vi "signal2.vi"() -> ()   [LabVIEW 2021]
panel:
  in  "?":bool
  out "Waveform Graph":dynamicdata(graph)
  in  "Noise Level 2":dbl(knob) scale=0.0..1.0
  in  "Amplitude 2":dbl(knob) scale=0.0..10.0
  in  "Frequency 2":dbl(knob) scale=0.0..10.0
  in  "Noise Level":dbl(knob) scale=0.0..1.0
  in  "Amplitude":dbl(knob) scale=0.0..10.0
  in  "Frequency":dbl(knob) scale=0.0..10.0
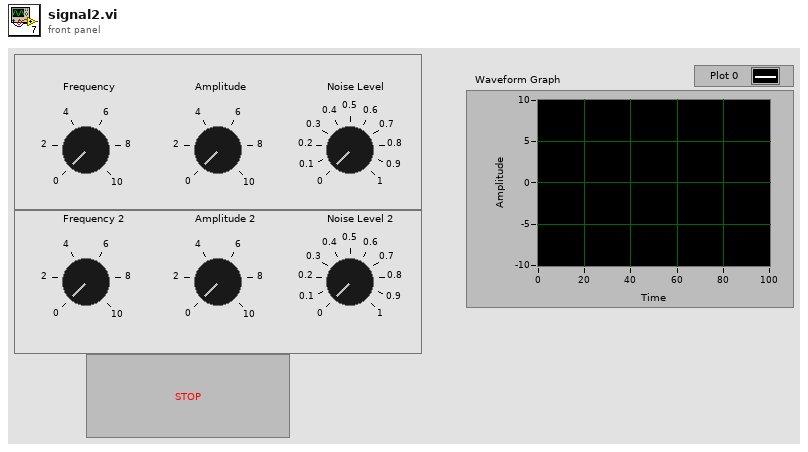
[diagram p1: front panel]
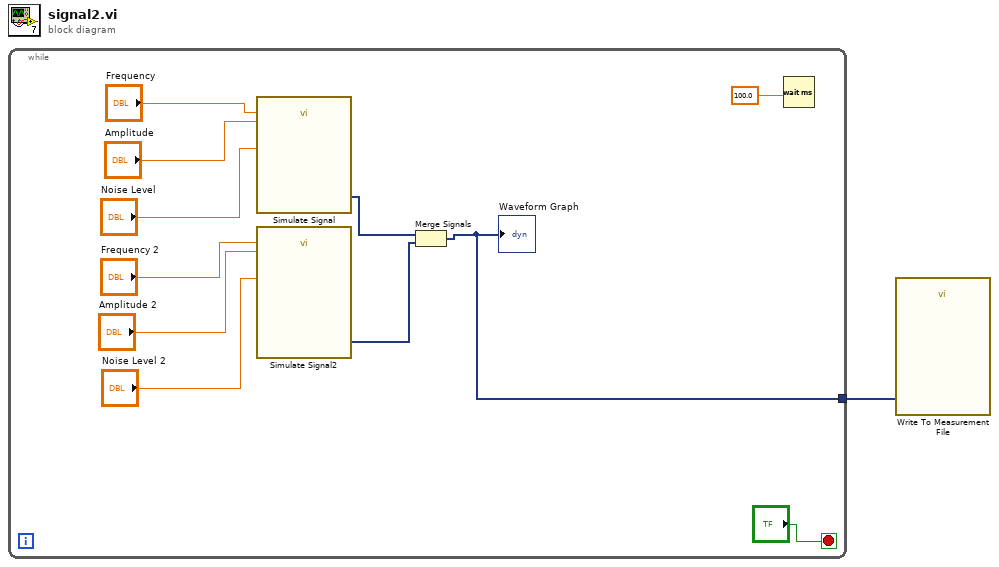
[diagram p0: block diagram]
diagram:
  n1 = while {
    tunnel: [w2] -> w1
    stop <- "?" stop-if-true
    n2 = call "Simulate Signal"("Frequency"="Frequency", "Amplitude"="Amplitude", "Standard deviation"="Noise Level") -> ("Sine with Gaussian Noise"=w6:dynamicdata)  [unwired: 11 in, 1 out]
    n3 = call "Simulate Signal2"("Frequency"="Frequency 2", "Amplitude"="Amplitude 2", "Standard deviation"="Noise Level 2") -> ("Sine with Gaussian Noise"=w5:dynamicdata)  [unwired: 11 in, 1 out]
    n4 = Merge Signals(w6, w5) -> (w2:dynamicdata)
    "Waveform Graph" <- w2
    n5 = Wait (ms)(milliseconds to wait=100.0) -> ()  [unwired: 1 out]
  }
  n6 = call "Write To Measurement File"("Signals"=w1) -> ()  [unwired: 16 in, 3 out]
